vi "svc_Spectrum Units.vi"(4 "error in (no error)":errorcluster, 6 "spectrum info in":T1={"channel name"="(Channel0)/(Channel0)", "description"="()/()", "x-axis units"=1, "spectral info"={"spectrum type"=enum."Frequency Response [Complex]", "linear/dB"=enum."linear", "window"=1, "window size"=512, "FFT size"=512}, "engineering units"=0, "custom label"="g/N", "dB reference [EU]"=1e-06, "peak units"=enum."rms", "weighting filter"=0, "spectral density?"=FALSE, "unit label"="", "spectrum skewed?"=FALSE, "complimentary spectrum units"=enum."radians"} {"x-axis units" items=["Time (s)"=0, "Frequency-CB (Hz)"=1, "Frequency-CPB (Hz)"=1248, "Frequency-Arbitrary (Hz)"=2357, "Quefrency (s)"=2, "Revolutions (rev)"=3, "Order"=4, "Speed (RPM)"=11, "Speed (rad/s)"=21, "Index"=65535]; "weighting filter" items=["Linear", "A-weighting", "B-weighting", "C-weighting", "ITU-R 468-4", "Dolby", "CCITT", "C-message", "Wb", "Wc", "Wd", "We", "Wf", "Wh", "Wj", "Wk", "Wm", "AES17 20 kHz lowpass", "AES17 40 kHz lowpass", "AES17 20 kHz highpass", "AES17 40 kHz highpass"]; "dB reference [EU]" format="%.2f"; "engineering units" items=["custom..."=0, "V"=1, "A"=21, "C"=30, "pC"=31, "s"=32, "-"=29, "Pa"=2, "N"=20, "g"=3, "m/s^2"=4, "m/s"=5, "m"=6, "mm/s"=12, "mm"=13, "micron/s"=14, "micron"=15, "in/s^2"=7, "in/s"=8, "in"=9, "mil/s"=10, "mil"=11, "rad/s^2"=16, "rad/s"=17, "rad"=18, "deg/s^2"=26, "deg/s"=27, "deg"=28, "RPM"=22, "cycle/s^2"=23, "Hz"=24, "cycle"=25, "strain"=19]; "spectral info"."window" items=["None "=0, "Hanning"=1, "Hamming"=2, "Blackman-Harris"=3, "Exact Blackman"=4, "Blackman"=5, "Flat Top"=6, "4 Term B-Harris "=7, "7 Term B-Harris"=8, "Low Sidelobe"=9, "Force - Exponential"=10, "Gaussian"=62]}) -> (0 "error out":errorcluster, 1 "x-axis unit label":string, 2 "spectrum info out":T1={"channel name"="(Channel0)/(Channel0)", "description"="()/()", "x-axis units"=1, "spectral info"={"spectrum type"=enum."Frequency Response [Complex]", "linear/dB"=enum."linear", "window"=1, "window size"=512, "FFT size"=512}, "engineering units"=0, "custom label"="g/N", "dB reference [EU]"=1e-06, "peak units"=enum."rms", "weighting filter"=0, "spectral density?"=FALSE, "unit label"="g/N|SV Units|dB ref 1.0E-6 g/N", "spectrum skewed?"=FALSE, "complimentary spectrum units"=enum."radians"} {"x-axis units" items=["Time (s)"=0, "Frequency-CB (Hz)"=1, "Frequency-CPB (Hz)"=1248, "Frequency-Arbitrary (Hz)"=2357, "Quefrency (s)"=2, "Revolutions (rev)"=3, "Order"=4, "Speed (RPM)"=11, "Speed (rad/s)"=21, "Index"=65535]; "weighting filter" items=["Linear", "A-weighting", "B-weighting", "C-weighting", "ITU-R 468-4", "Dolby", "CCITT", "C-message", "Wb", "Wc", "Wd", "We", "Wf", "Wh", "Wj", "Wk", "Wm", "AES17 20 kHz lowpass", "AES17 40 kHz lowpass", "AES17 20 kHz highpass", "AES17 40 kHz highpass"]; "dB reference [EU]" format="%.2f"; "engineering units" items=["custom..."=0, "V"=1, "A"=21, "C"=30, "pC"=31, "s"=32, "-"=29, "Pa"=2, "N"=20, "g"=3, "m/s^2"=4, "m/s"=5, "m"=6, "mm/s"=12, "mm"=13, "micron/s"=14, "micron"=15, "in/s^2"=7, "in/s"=8, "in"=9, "mil/s"=10, "mil"=11, "rad/s^2"=16, "rad/s"=17, "rad"=18, "deg/s^2"=26, "deg/s"=27, "deg"=28, "RPM"=22, "cycle/s^2"=23, "Hz"=24, "cycle"=25, "strain"=19]; "spectral info"."window" items=["None "=0, "Hanning"=1, "Hamming"=2, "Blackman-Harris"=3, "Exact Blackman"=4, "Blackman"=5, "Flat Top"=6, "4 Term B-Harris "=7, "7 Term B-Harris"=8, "Low Sidelobe"=9, "Force - Exponential"=10, "Gaussian"=62]}, 3 "unit label":string)   [LabVIEW 2017]
doc: "This VI generates unit labels from spectrum info. Unit labels are created for both linear and dB units and returned in unit label string. Subsequent calls to this VI will check if unit label has already been generated and extract appropriate unit label based on linear/dB field in spectrum info. \n\nGeneral Rule - If you change the spectrum, change spectrum info. If you change spectrum info, clear the unit label field so that correct units will be generated downstream.\nException - Changing linear/dB does not force you to clear unit label field as both strings are generated."
uses:
  <vilib>/addons/_NISVFA/_Shared subVIs/Controls/svc_Spectrum Info.ctl
  <vilib>/addons/_NISVFA/_Shared subVIs/Controls/svc_X-Axis Units.ctl
  <vilib>/addons/_NISVFA/_Shared subVIs/Controls/svc_Spectrum Type.ctl
  <vilib>/addons/_NISVFA/_Shared subVIs/Controls/svc_Engineering Units Text Ring.ctl
  <vilib>/addons/_NISVFA/_Shared subVIs/Controls/svc_Weighting Filter Text Ring.ctl
  <vilib>/addons/_NISVFA/_Shared subVIs/Controls/svc_Complimentary Spectrum Units.ctl
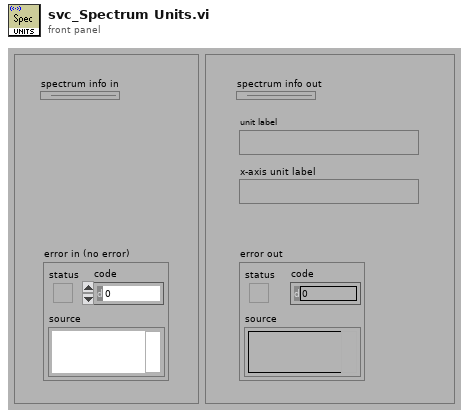
[diagram p1: front panel]
types:
  T1 = typedef "svc_Spectrum Info.ctl" = cluster{"channel name":string, "description":string, "x-axis units":T2, "spectral info":cluster{"spectrum type":T3, "linear/dB":enum16{"linear", "dB"}, "window":u16, "window size":i32, "FFT size":i32}, "engineering units":T4, "custom label":string, "dB reference [EU]":dbl, "peak units":enum16{"rms", "peak", "peak-peak"}, "weighting filter":T5, "spectral density?":bool, "unit label":string, "spectrum skewed?":bool, "complimentary spectrum units":T6}
  T2 = typedef "svc_X-Axis Units.ctl" = u16
  T3 = typedef "svc_Spectrum Type.ctl" = enum16{"FFT Spectrum [complex]", "Amplitude [Magnitude]", "Power [Magnitude^2]", "Cross Spectrum [complex]", "Frequency Response [Complex]"}
  T4 = typedef "svc_Engineering Units Text Ring.ctl" = u16
  T5 = typedef "svc_Weighting Filter Text Ring.ctl" = u16
  T6 = typedef "svc_Complimentary Spectrum Units.ctl" = enum16{"none", "radians", "degrees", "cycles", "imaginary"}
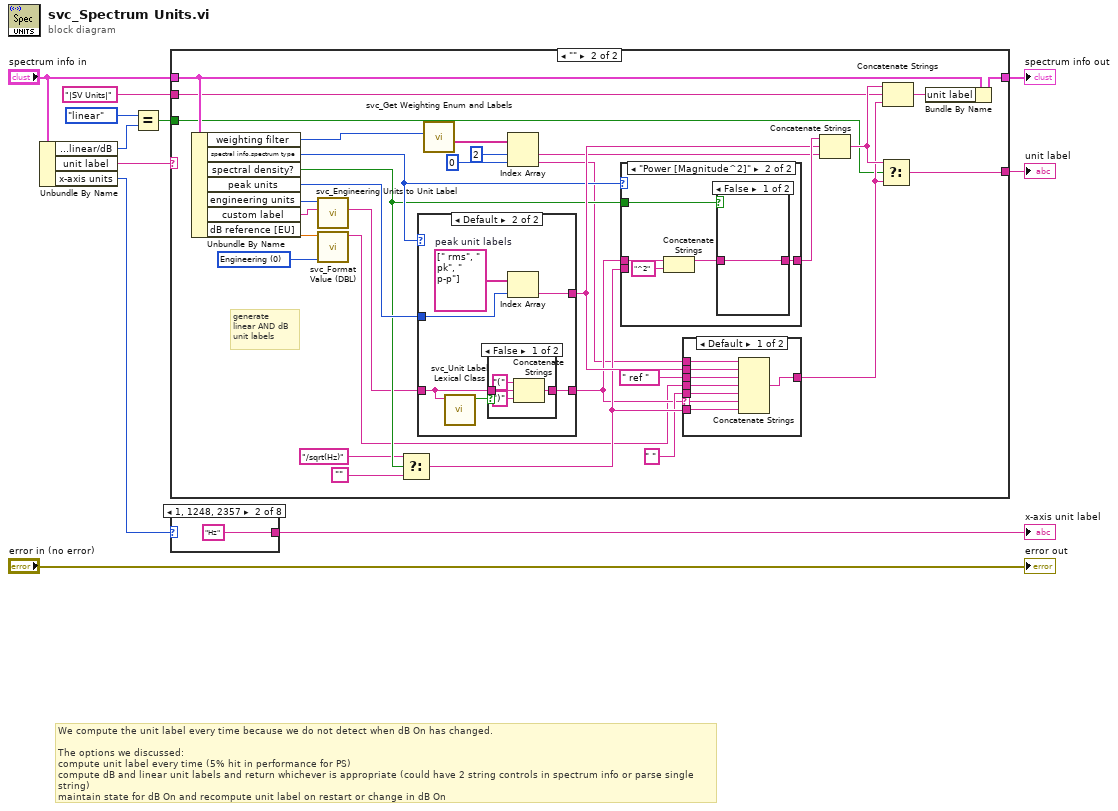
[diagram p0: block diagram]
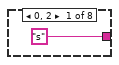
[diagram p2: hidden frame]
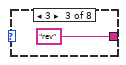
[diagram p3: hidden frame]
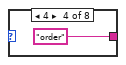
[diagram p4: hidden frame]
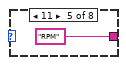
[diagram p5: hidden frame]
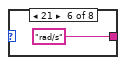
[diagram p6: hidden frame]
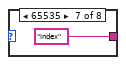
[diagram p7: hidden frame]
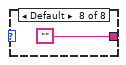
[diagram p8: hidden frame]
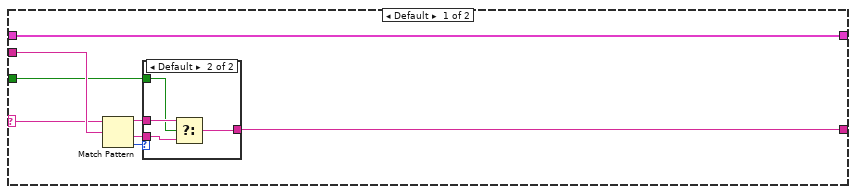
[diagram p9: hidden frame]
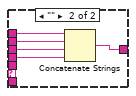
[diagram p11: hidden frame]
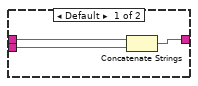
[diagram p12: hidden frame]
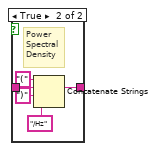
[diagram p13: hidden frame]
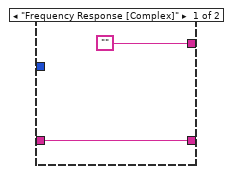
[diagram p14: hidden frame]
diagram:
  # "We compute the unit label every time because we do not detect when dB On has changed.\n\nThe options we discussed:\ncompute unit label every time (5% hit in performance for PS)\ncompute dB and linear unit labels and return whichever is appropriate (could have 2 string controls in spectrum info or parse single string)\nmaintain state for dB On and recompute unit label on restart or change in dB On"
  n1 = Unbundle By Name("spectrum info in") -> ("spectral info.linear/dB"=w2:enum16{"linear", "dB"}, "unit label"=w5:string, "x-axis units"=w6:T2)
  n2 = Equal?(x=enum16{"linear", "dB"}."linear" ("y"), y=w2) -> (x = y?=w1:bool)
  n3 = case shown="\"\"" w5 {
    selector: w5 -> [w13 _]
    tunnel: [w16 w52] -> w10
    tunnel: "spectrum info in" -> [w14 w53]
    tunnel: [w14 w54] -> w9
    tunnel: "|SV Units|" ("string") -> [w19 w47]
    tunnel: w1 -> [w12 w31]
    frame Default {
      n4 = Match Pattern(string=w13, regular expression=w19) -> (before substring=w18:string, after substring=w17:string, offset past match=w15:i32)  [unwired: 1 in, 1 out]
      n5 = case shown="Default" w15 {
        tunnel: w18 -> [w20 w24]
        tunnel: w17 -> [_ w23]
        tunnel: [w20 w22] -> w16
        tunnel: w12 -> [_ w21]
        frame -1 {
        }
        frame Default {
          n6 = Select(t=w24, s=w21, f=w23) -> (s? t:f=w22:string)
        }
      }
    }
    frame "" {
      w25 = i16 0 items=["Engineering", "Exponential", "Fractional", "Automatic"] ("number format")
      # "generate \nlinear AND dB\nunit labels"
      n7 = Unbundle By Name(w53) -> ("weighting filter"=w45:T5, "spectral info.spectrum type"=w41:T3, "spectral density?"=w39:bool, "peak units"=w55:enum16{"rms", "peak", "peak-peak"}, "engineering units"=w43:T4, "custom label"=w42:string, "dB reference [EU]"=w34:dbl)
      n8 = call <vilib>:"svc_Engineering Units to Unit Label.vi"("custom label"=w42, "engineering units"=w43) -> ("unit label"=w33:string)  [unwired: 8 in, 1 out]
      n9 = call <vilib>:"svc_Format Value (DBL).vi"("number format"=w25, "dB reference"=w34) -> ("format string"=w30:string)  [unwired: 9 in]
      n10 = Select(t="/sqrt(Hz)" ("resulting unit label"), s=w39, f="") -> (s? t:f=w36:string)
      n11 = case shown="Default" w41 {
        tunnel: ["" ("Empty String Constant") w88] -> w46
        tunnel: w55 -> [_ w90]
        tunnel: w33 -> [w83 w86]
        tunnel: [w83 w85] -> w32
        frame "Frequency Response [Complex]" {
        }
        frame Default {
          w89 = string[] [" rms", " pk", " p-p"]  # peak unit labels
          n12 = call <vilib>:"svc_Unit Label Lexical Class.vi"("unit label"=w86) -> ("letters only?"=w87:bool)  [unwired: 6 in]
          n13 = case shown="False" w87 {
            tunnel: w86 -> [w94 w95]
            tunnel: [w93 w95] -> w85
            frame False {
              n14 = Concatenate Strings("(" ("string"), w94, ")" ("string")) -> (w93:string)
            }
            frame True {
            }
          }
          n15 = Index Array(array=w89, index=w90) -> (element=w88:string)
        }
      }
      n16 = call <vilib>:"svc_Get Weighting Enum and Labels.vi"("weighting filter"=w45) -> ("weighting subarray"=w44:string[])  [unwired: 7 in, 1 out]
      n17 = Index Array(array=w44, index #1=2 ("index"), index #2=0 ("index")) -> (element #1=w27:string, element #2=w26:string)
      n18 = case shown="\"Power [Magnitude^2]\"" w41 {
        tunnel: [w69 w75] -> w48
        tunnel: w39 -> [_ w76]
        tunnel: w32 -> [w70 w72]
        tunnel: w36 -> [w71 _]
        frame Default {
          n19 = Concatenate Strings(w70, w71) -> (w69:string)
        }
        frame "Power [Magnitude^2]" {
          n20 = Concatenate Strings(w72, "^2") -> (w74:string)
          n21 = case shown="False" w76 {
            tunnel: w74 -> [w77 w81]
            tunnel: [w77 w82] -> w75
            frame False {
            }
            frame True {
              # "Power\nSpectral\nDensity"
              n22 = Concatenate Strings("(" ("Substring"), w81, ")" ("Substring"), "/Hz" ("resulting unit label")) -> (w82:string)
            }
          }
        }
      }
      n23 = case shown="Default" w32 {
        selector: w32 -> [w59 _]
        tunnel: [w63 w68] -> w50
        tunnel: w26 -> [w62 w67]
        tunnel: w30 -> [w61 w66]
        tunnel: w46 -> [w60 w65]
        tunnel: " ref " ("string") -> [w58 w64]
        tunnel: w36 -> [w57 _]
        tunnel: " " ("Substring") -> [w56 _]
        frame Default {
          n24 = Concatenate Strings(w62, w60, w58, w61, w56, w59, w57) -> (w63:string)
        }
        frame "" {
          n25 = Concatenate Strings(w67, w65, w64, w66) -> (w68:string)
        }
      }
      n26 = Concatenate Strings(w48, w46, w27) -> (w51:string)
      n27 = Select(t=w51, s=w31, f=w50) -> (s? t:f=w52:string)
      n28 = Concatenate Strings(w51, w47, w50) -> (w49:string)
      n29 = Bundle By Name(cluster=w53, "unit label"=w49) -> (w54:T1)
    }
  }
  "spectrum info out" <- w9
  "unit label" <- w10
  n30 = case shown="1, 1248, 2357" w6 {
    tunnel: ["s" "Hz" "rev" "order" "RPM" "rad/s" "index" "" ("Empty String Constant")] -> w8
    frame 0, 2 {
    }
    frame 1, 1248, 2357 {
    }
    frame 3 {
    }
    frame 4 {
    }
    frame 11 {
    }
    frame 21 {
    }
    frame 65535 {
    }
    frame Default {
    }
  }
  "x-axis unit label" <- w8
  "error out" <- "error in (no error)"
